vi "LVM.vi"(8 "dy":dbl, 9 "dx":dbl, 10 "Phase":i32, 11 "Dir":i32) -> ()   [LabVIEW 2014]
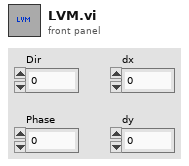
[diagram p1: front panel]
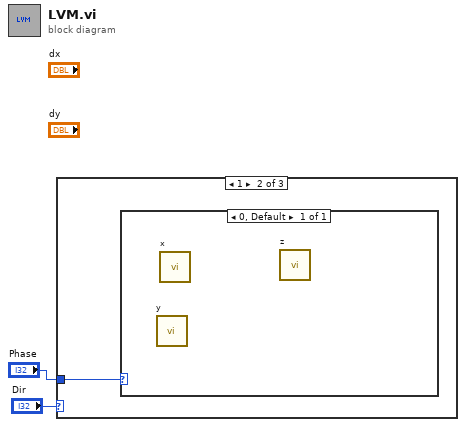
[diagram p0: block diagram]
diagram:
  n1 = case shown="1" "Dir" {
    tunnel: "Phase" -> [w3 w4 w5]
    frame 0, Default {
      n2 = case shown="1" w3 {
        frame 0, Default {
        }
        frame 1 {
        }
      }
    }
    frame 1 {
      n3 = case shown="0, Default" w4 {
        frame 0, Default {
          n4 = call "y"() -> ()  [unwired: 9 in, 3 out]
          n5 = call "x"() -> ()  [unwired: 9 in, 3 out]
          n6 = call "z"() -> ()  [unwired: 9 in, 3 out]
        }
      }
    }
    frame 2 {
      n7 = case shown="1" w5 {
        frame 0, Default {
        }
        frame 1 {
        }
      }
    }
  }
